vi "PQlistTables.vi"(8 "error in":errorcluster, 11 "conn":u64) -> (0 "error out":errorcluster, 2 "Data":string[](array[string]), 3 "conn_out":u64)   [LabVIEW 2019, in "libpqutility64.lvlib"]
uses:
  libpqutility64.lvlib
  libpqlv64/src/PQgetResult.vi
  libpqlv64/src/PQclear.vi
  PQfetchTables.vi
  libpqlv64/src/PQresultErrorMessage.vi
  libpqlv64/src/PQresultStatus.vi
  libpqlv64/src/PQsendQuery.vi
  libpqlv64/src/PQgetvalue.vi
  libpqlv64/src/PQntuples.vi
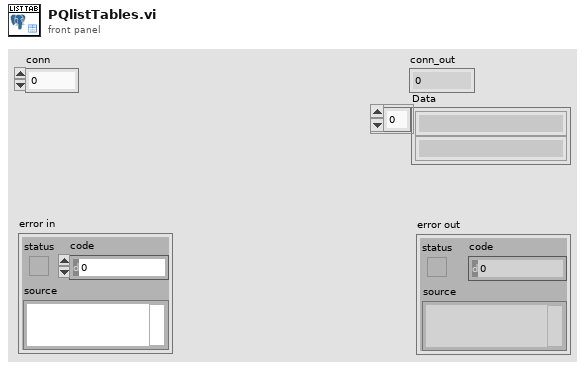
[diagram p1: front panel]
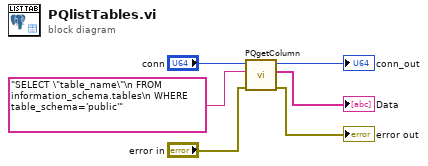
[diagram p0: block diagram]
diagram:
  n1 = call "PQgetColumn.vi"("error in"="error in", "query"="SELECT \"table_name\"\n FROM information_schema.tables\n WHERE table_schema='public'", "conn"="conn") -> ("error out"=→"error out":errorcluster, "Data"=→"Data":string[], "conn_out"=→"conn_out":u64)  [unwired: 6 in]
